vi "SetAxisParameterString.vi"(0 "Controller In":refnum<k24>, 5 "axisName":string, 7 "Parameter Name":string(combo), 9 "value":string, 11 "error in (no error)":errorcluster) -> (4 "Controller Out":refnum<k24>, 15 "error out":errorcluster)   [LabVIEW 2021]
uses:
  C:/Program Files (x86)/Aerotech/A3200/LabVIEW/2010/Bin/Aerotech.A3200.dll
  Bin/Aerotech.A3200.dll
  C:/Program Files (x86)/Aerotech/A3200/LabVIEW/2010/Bin/Aerotech.A3200.LabVIEW.dll
  Bin/Aerotech.A3200.LabVIEW.dll
panel:
  out "ParameterType":i32(ring)=4 items=["Integer", "Double", "Single", "Long", "String"]
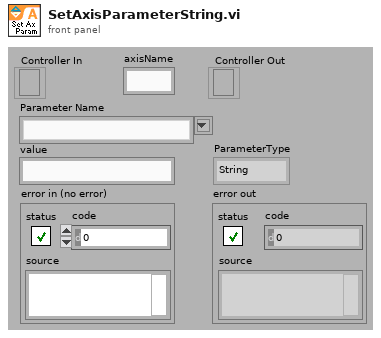
[diagram p1: front panel]
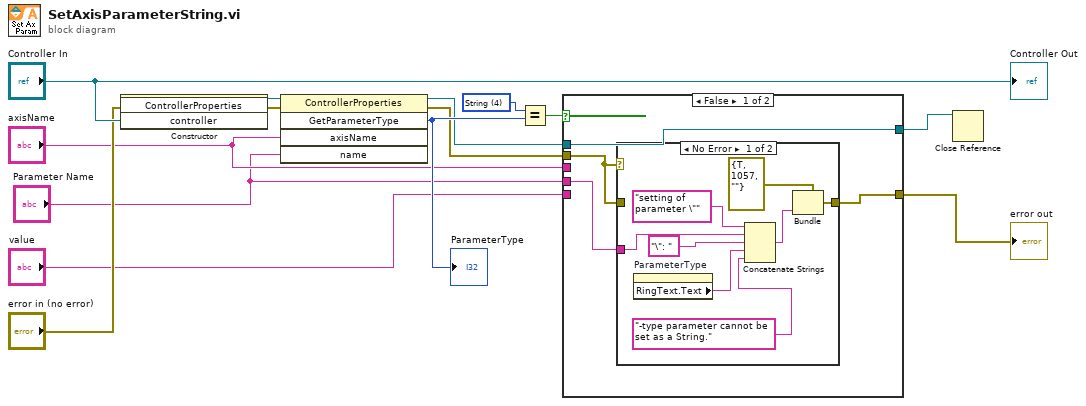
[diagram p0: block diagram]
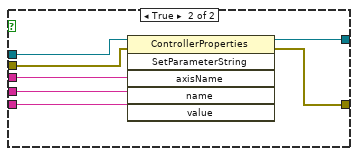
[diagram p3: hidden frame]
diagram:
  w10 = 4 items=["Integer", "Double", "Single", "Long", "String"] ("GetParameterType")
  n1 = constructor class="ControllerProperties"(error in="error in (no error)", "controller"="Controller In") -> (reference out=w12:refnum<k24>, error out=w11:errorcluster)  [unwired: 2 in, 2 out]
  n2 = invoke class="ControllerProperties" method="GetParameterType"(reference=w12, error in=w11, "axisName"="axisName", "name"="Parameter Name") -> (reference out=w6:refnum<k24>, error out=w5:errorcluster, "GetParameterType"=w9:i32)  [unwired: 1 in, 2 out]
  "ParameterType" <- w9
  n3 = Equal?(x=w10, y=w9) -> (x = y?=w8:bool)
  n4 = case shown="False" w8 {
    tunnel: [w18 w33] -> w7
    tunnel: w6 -> [w18 w34]
    tunnel: "Parameter Name" -> [w15 w30]
    tunnel: w5 -> [w16 w32]
    tunnel: [w17 w31] -> w4
    tunnel: "axisName" -> [_ w29]
    tunnel: "value" -> [_ w28]
    frame False {
      n5 = case shown="No Error" w16 {
        tunnel: [w25 w27] -> w17
        tunnel: w16 -> [_ w27]
        tunnel: w15 -> [w22 _]
        frame No Error {
          n6 = property on="ParameterType" class="Ring (strict)"() -> ("RingText.Text"=w20:string)  [unwired: 2 in, 2 out]
          n7 = Concatenate Strings("setting of parameter \"" ("string"), w22, "\": " ("string"), w20, "-type parameter cannot be set as a String." ("string")) -> (w24:string)
          n8 = Bundle(cluster=cluster{bool, "code":i32, "source":string} {TRUE, "code"=1057, "source"=""} ("error out"), "source"=w24) -> (w25:cluster{bool, "code":i32, "source":string})  [unwired: 2 in]
        }
        frame Error {
        }
      }
    }
    frame True {
      n9 = invoke class="ControllerProperties" method="SetParameterString"(reference=w34, error in=w32, "axisName"=w29, "name"=w30, "value"=w28) -> (reference out=w33:refnum<k24>, error out=w31:errorcluster)  [unwired: 1 in, 4 out]
    }
  }
  "error out" <- w4
  n10 = Close Reference(reference=w7) -> ()  [unwired: 1 in, 1 out]
  "Controller Out" <- "Controller In"
